vi "Лабораторная №1 Задание 3_1.vi"() -> ()   [LabVIEW 2017]
panel:
  out "Product":dbl
  out "Sum":dbl
  in  "Knob":dbl(knob) scale=0.0..10.0
  in  "Slide":dbl(slide) scale=0.0..10.0
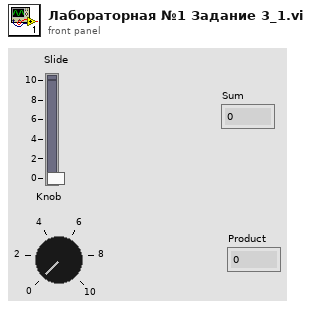
[diagram p1: front panel]
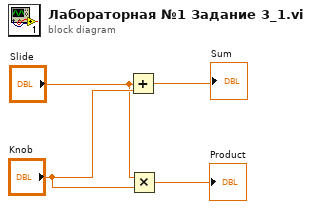
[diagram p0: block diagram]
diagram:
  n1 = Add(x="Slide", y="Knob") -> (x+y=→"Sum":dbl)
  n2 = Multiply(x="Slide", y="Knob") -> (x*y=→"Product":dbl)
